vi "Append Timeout.vi"(0 "Tosca in":refnum<class "Parameters.lvclass">, 5 "Timeout":refnum<class "Timeout.lvclass">, 7 "stateIndex":i32, 11 "error in (no error)":errorcluster) -> (4 "Tosca out":refnum<class "Parameters.lvclass">, 15 "error out":errorcluster)   [LabVIEW 2015, in "Parameters.lvclass"]
uses:
  Parameters.lvclass
  Timeout/Timeout.lvclass
  Parameters.lvclass/Parameters.ctl
  State/State.lvclass
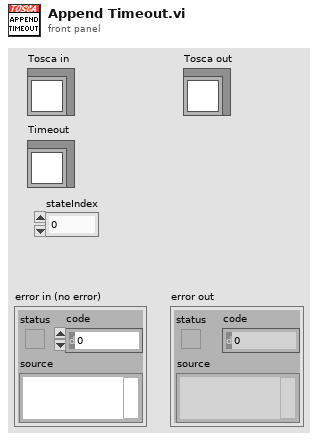
[diagram p1: front panel]
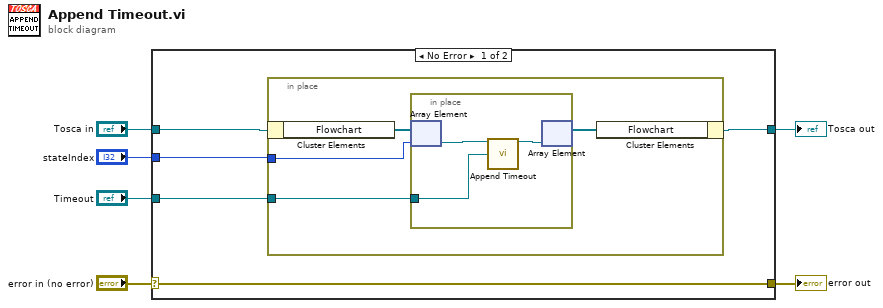
[diagram p0: block diagram]
diagram:
  n1 = case shown="No Error" "error in (no error)" {
    selector: "error in (no error)" -> [w11 w20]
    tunnel: [w11 w20] -> w5
    tunnel: [w9 w19] -> w3
    tunnel: "Tosca in" -> [w10 w19]
    tunnel: "stateIndex" -> [w8 _]
    tunnel: "Timeout" -> [w7 _]
    frame No Error {
      n2 = in-place {
        in-place-border: w8 -> [w14]
        in-place-border: w7 -> [w12]
        n3 = in-place-cluster #1(w10) -> ("Flowchart"=w15:refnum<class "State.lvclass">[])
        n4 = in-place {
          in-place-border: w12 -> [w16]
          n5 = in-place-array #2(w15, w14) -> (w18:refnum<class "State.lvclass">)
          n6 = call "Append Timeout.vi"("State in"=w18, "Timeout"=w16) -> ("State out"=w17:refnum<class "State.lvclass">)  [unwired: 12 in, 1 out]
          n7 = in-place-array #2(w17) -> (w13:refnum<class "State.lvclass">[])  [unwired: 1 out]
        }
        n8 = in-place-cluster #1("Flowchart"=w13) -> (w9:refnum<class "Parameters.lvclass">)
      }
    }
    frame Error {
    }
  }
  "error out" <- w5
  "Tosca out" <- w3
